vi "DIO_ActionEngine.vi"(8 "error in":errorcluster, 9 "System Outputs":bool[](array[boolean]), 10 "Clock":bool, 11 "DIO Action":T1) -> (0 "error out":errorcluster, 2 "System Inputs":bool[](array[boolean]), 3 "Reset":bool)   [LabVIEW 2018]
uses:
  DIO_Action(enum).ctl
  <vilib>/DAQmx/read.llb/DAQmx Read (Digital 1D Bool 1Chan 1Samp).vi
  <vilib>/DAQmx/read.llb/DAQmx Read (Analog DBL 1Chan 1Samp).vi
  <vilib>/DAQmx/write.llb/DAQmx Write (Digital 1D Bool 1Chan 1Samp).vi
  <vilib>/DAQmx/write.llb/DAQmx Write (Analog DBL 1Chan 1Samp).vi
  <vilib>/DAQmx/create/channels.llb/DAQmx Create Channel (DI-Digital Input).vi
  <vilib>/DAQmx/create/channels.llb/DAQmx Create Channel (DO-Digital Output).vi
  <vilib>/DAQmx/create/channels.llb/DAQmx Create Channel (AI-Voltage-Basic).vi
  <vilib>/DAQmx/create/channels.llb/DAQmx Create Channel (AO-Voltage-Basic).vi
  <vilib>/DAQmx/miscellaneous.llb/DAQmx Fill In Error Info.vi
panel:
  # "Locked"
  # "B3"
  # "C"
  # "B2"
  # "B"
  # "B1"
  # "A"
  # "B0"
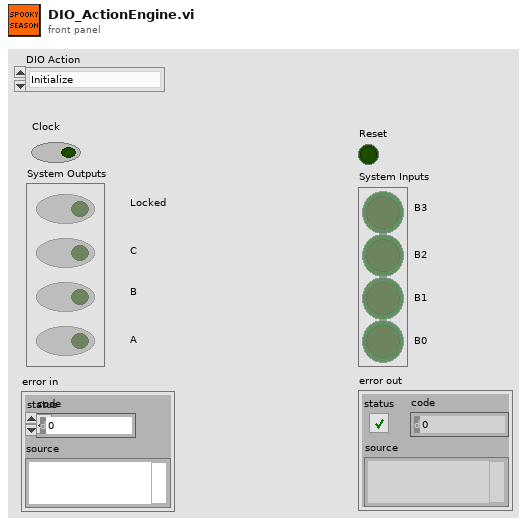
[diagram p1: front panel]
types:
  T1 = typedef "DIO_Action(enum).ctl" = enum16{"Initialize", "Read Code Entry Buttons", "Read Reset Button", "Write Lock Status", "Write Clock", "Release"}
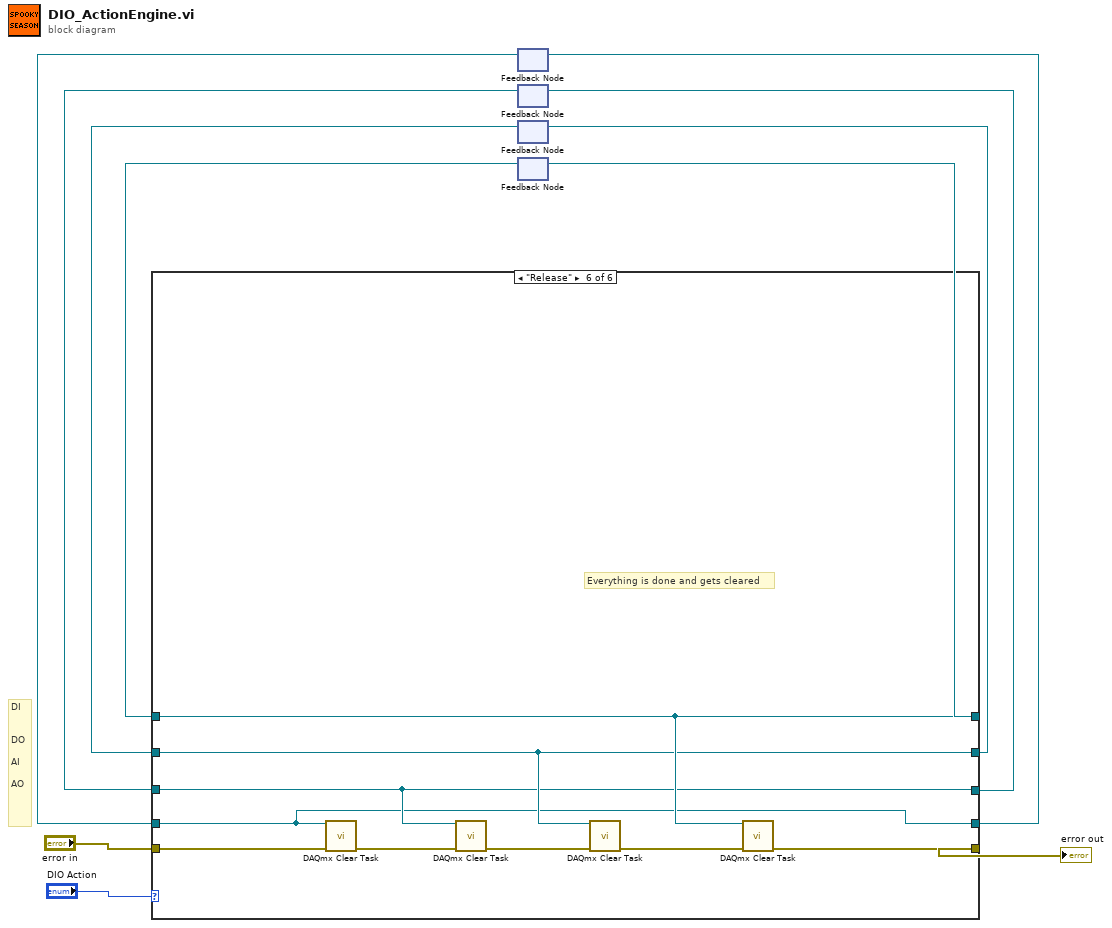
[diagram p0: block diagram]
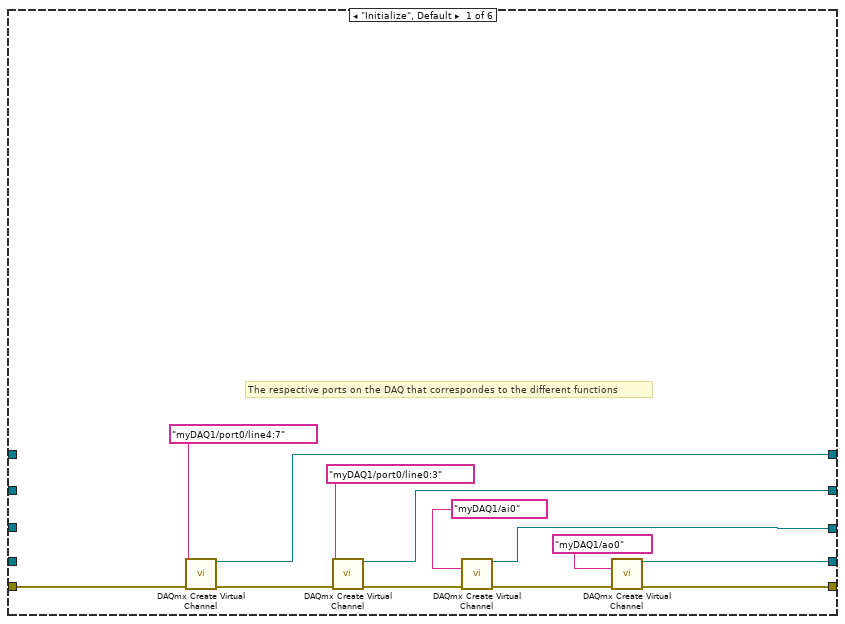
[diagram p2: hidden frame]
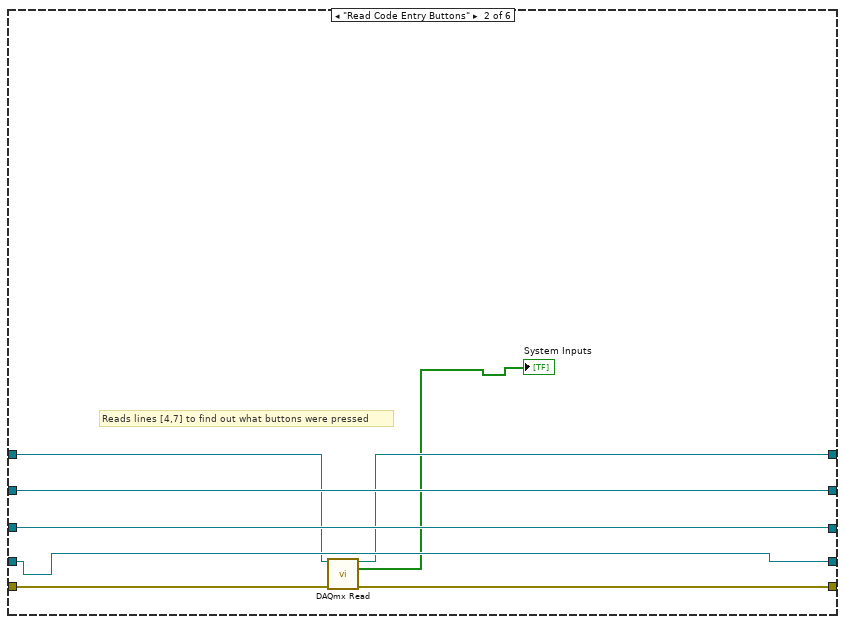
[diagram p3: hidden frame]
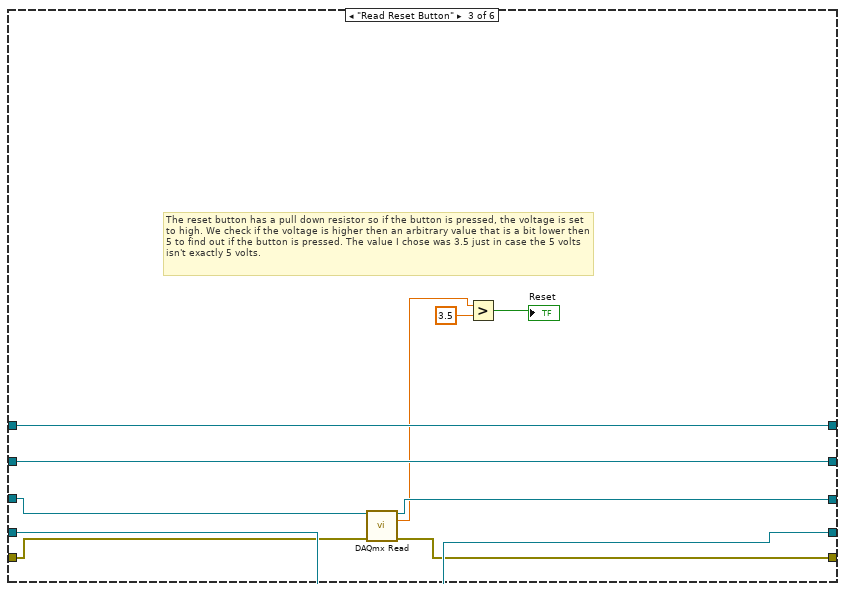
[diagram p4: hidden frame]
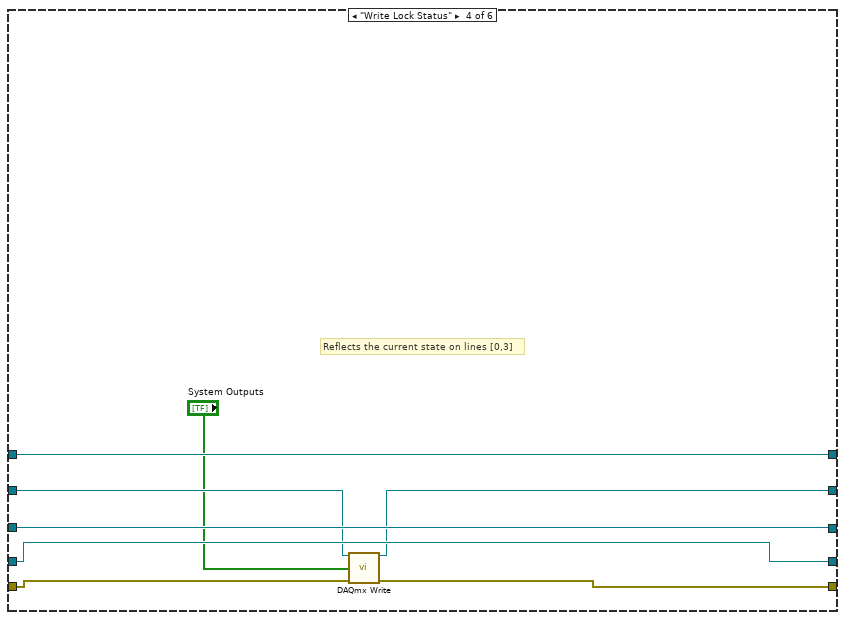
[diagram p5: hidden frame]
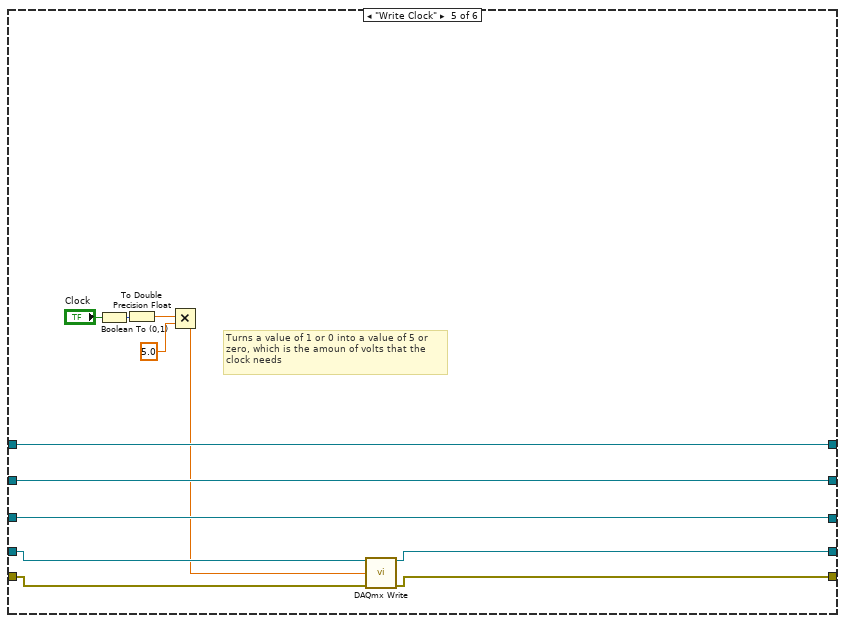
[diagram p6: hidden frame]
diagram:
  # "DI\n\n\nDO\n\nAI\n\nAO"
  n1 = feedback #1() -> (w1:refnum<k21>)  [unwired: 1 in]
  n2 = feedback #2() -> (w2:refnum<k21>)  [unwired: 1 in]
  n3 = feedback #3() -> (w3:refnum<k21>)  [unwired: 1 in]
  n4 = feedback #4() -> (w4:refnum<k21>)  [unwired: 1 in]
  n5 = case shown="\"Release\"" "DIO Action" {
    tunnel: "error in" -> [w24 w32 w34 w50 w62 w71]
    tunnel: [w20 w31 w33 w49 w61 w67] -> w9
    tunnel: [w19 w30 w40 w46 w59 w63] -> w8
    tunnel: [w18 w29 w38 w47 w58 w64] -> w7
    tunnel: [w17 w28 w41 w44 w57 w65] -> w6
    tunnel: [w16 w26 w42 w48 w56 w66] -> w5
    tunnel: w4 -> [_ w27 w42 w48 w56 w66]
    tunnel: w3 -> [_ w28 w41 w45 w57 w65]
    tunnel: w2 -> [_ w29 w39 w47 w58 w64]
    tunnel: w1 -> [_ w30 w40 w46 w60 w63]
    frame "Initialize", Default {
      # "The respective ports on the DAQ that correspondes to the different functions"
      n6 = call-poly <vilib>:"DAQmx Create Virtual Channel.vi"("lines"=tag "myDAQ1/port0/line4:7", "error in"=w24) -> ("task out"=w16:refnum<k21>, "error out"=w23:errorcluster)  [unwired: 12 in]
      n7 = call-poly <vilib>:"DAQmx Create Virtual Channel.vi"("lines"=tag "myDAQ1/port0/line0:3", "error in"=w23) -> ("task out"=w17:refnum<k21>, "error out"=w22:errorcluster)  [unwired: 12 in]
      n8 = call-poly <vilib>:"DAQmx Create Virtual Channel.vi"("physical channels"=tag "myDAQ1/ai0", "error in"=w22) -> ("task out"=w18:refnum<k21>, "error out"=w21:errorcluster)  [unwired: 12 in]
      n9 = call-poly <vilib>:"DAQmx Create Virtual Channel.vi"("physical channels"=tag "myDAQ1/ao0", "error in"=w21) -> ("task out"=w19:refnum<k21>, "error out"=w20:errorcluster)  [unwired: 12 in]
    }
    frame "Read Code Entry Buttons" {
      # "Reads lines [4,7] to find out what buttons were pressed"
      n10 = call-poly <vilib>:"DAQmx Read.vi"("task/channels in"=w27, "error in"=w32) -> ("task out"=w26:refnum<k21>, "data"=→"System Inputs":bool[], "error out"=w31:errorcluster)  [unwired: 11 in]
    }
    frame "Read Reset Button" {
      # "The reset button has a pull down resistor so if the button is pressed, the voltage is set to high. We check if the voltage is higher then an arbitrary value that is a bit lower then 5 to find out if the button is pressed. The value I chose was 3.5 just in case the 5 volts isn't exactly 5 volts."
      n11 = call-poly <vilib>:"DAQmx Read.vi"("task/channels in"=w39, "error in"=w34) -> ("task out"=w38:refnum<k21>, "data"=w36:dbl, "error out"=w33:errorcluster)  [unwired: 11 in]
      n12 = Greater?(x=w36, y=3.5) -> (0:→"Reset":bool)
    }
    frame "Write Lock Status" {
      # "Reflects the current state on lines [0,3]"
      n13 = call-poly <vilib>:"DAQmx Write.vi"("task/channels in"=w45, "data"="System Outputs", "error in"=w50) -> ("task out"=w44:refnum<k21>, "error out"=w49:errorcluster)  [unwired: 10 in, 1 out]
    }
    frame "Write Clock" {
      # "Turns a value of 1 or 0 into a value of 5 or zero, which is the amoun of volts that the clock needs"
      n14 = Boolean To (0,1)(Boolean="Clock") -> (0, 1=w54:i16)
      n15 = To Double Precision Float(number=w54) -> (double precision float=w53:dbl)
      n16 = Multiply(x=w53, y=5.0) -> (x*y=w51:dbl)
      n17 = call-poly <vilib>:"DAQmx Write.vi"("task/channels in"=w60, "data"=w51, "error in"=w62) -> ("task out"=w59:refnum<k21>, "error out"=w61:errorcluster)  [unwired: 10 in, 1 out]
    }
    frame "Release" {
      # "Everything is done and gets cleared"
      n18 = call <vilib>:"DAQmx Clear Task.vi"("task in"=w63, "error in"=w71) -> ("error out"=w70:errorcluster)  [unwired: 13 in]
      n19 = call <vilib>:"DAQmx Clear Task.vi"("task in"=w64, "error in"=w70) -> ("error out"=w69:errorcluster)  [unwired: 13 in]
      n20 = call <vilib>:"DAQmx Clear Task.vi"("task in"=w65, "error in"=w69) -> ("error out"=w68:errorcluster)  [unwired: 13 in]
      n21 = call <vilib>:"DAQmx Clear Task.vi"("task in"=w66, "error in"=w68) -> ("error out"=w67:errorcluster)  [unwired: 13 in]
    }
  }
  "error out" <- w9
  n22 = feedback-in #1(w8) -> ()
  n23 = feedback-in #2(w7) -> ()
  n24 = feedback-in #3(w6) -> ()
  n25 = feedback-in #4(w5) -> ()
